vi "StartNewErrorLog.vi"(7 "LabVIEW Web Service Request":refnum<class "Web Request.lvclass">) -> ()   [LabVIEW 2018]
uses:
  <vilib>/wsapi/Web Request.lvclass
  CAEN globals.vi
panel:
  in  "error in (no error)":errorcluster
  # "Use the Web Service Request input terminal to call the VIs on the Web Services palette. Do not remove it from the connector pane unless you don't need access to the palette."
  # "Each additional control wired to the connector pane will be available as an input in the URL. To include an indicator in terminal-mode output (the default setting), it must also be wired to the connector pane."
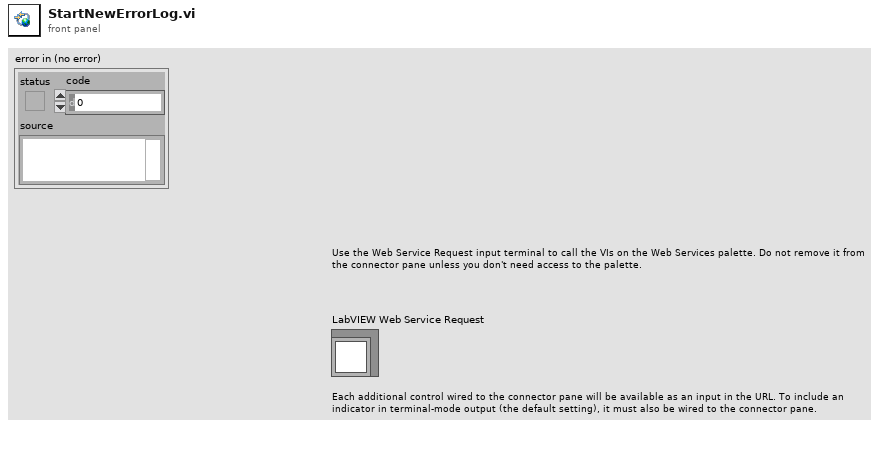
[diagram p1: front panel]
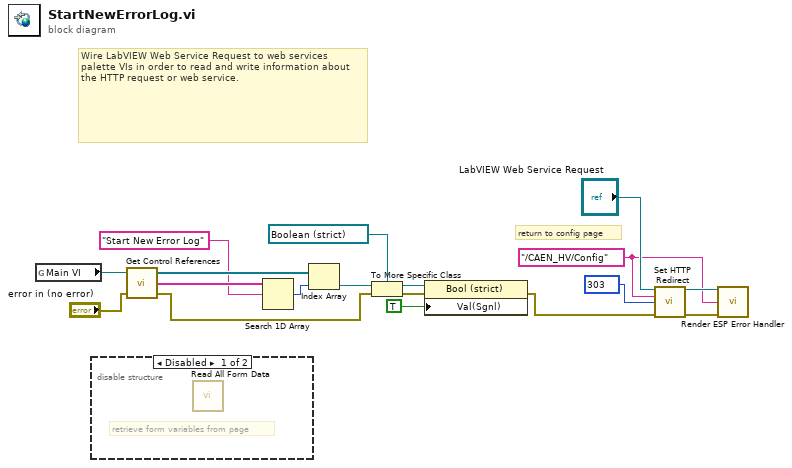
[diagram p0: block diagram]
diagram:
  w6 = 303 items=["100"=100, "101"=101, "200"=200, "201"=201, "202"=202, "203"=203, "204"=204, "205"=205, "206"=206, "300"=300, "301"=301, "302"=302, "303"=303, "304"=304, "305"=305, "306"=306, "307"=307, "400"=400, "401"=401, "402"=402, "403"=403, "404"=404, "405"=405, "406"=406, "407"=407, "408"=408, "409"=409, "410"=410, "411"=411, "412"=412, "413"=413, "414"=414, "415"=415, "416"=416, "417"=417, "500"=500, "501"=501, "502"=502, "503"=503, "504"=504, "505"=505] ("response code (307)")
  w1 = "/CAEN_HV/Config" ("redirect URL")
  # "return to config page"
  # "Wire LabVIEW Web Service Request to web services palette VIs in order to read and write information about the HTTP request or web service."
  n1 = global read "CAEN globals.vi" "Main VI"() -> (w18:refnum<vi>)
  n2 = disable-structure shown="Disabled" {
    frame Disabled {
      # "retrieve form variables from page"
      n3 = call <vilib>:"Read All Form Data.vi"() -> ()  [unwired: 11 in, 5 out]
    }
    frame Enabled {
    }
  }
  n4 = call "Get Control References.vi"("error in"="error in (no error)", "This vi"=w18) -> ("error out"=w8:errorcluster, "Control Names"=w17:string[], "Controls[]"=w16:refnum<vi>[])  [unwired: 1 in]
  n5 = Search 1D Array(1D array=w17, element="Start New Error Log" ("Label.Text")) -> (index of element=w11:i32)  [unwired: 1 in]
  n6 = Index Array(array=w16, index=w11) -> (element=w9:refnum<vi>)
  n7 = To More Specific Class(target class=refnum<vi> refnum ("replace all? (F)"), reference=w9, error in=w8) -> (specific class reference=w13:refnum<vi>, error out=w14:errorcluster)
  n8 = property class="Bool (strict)"(reference=w13, error in=w14, "Val(Sgnl)"=TRUE ("Value (Signaling)")) -> (error out=w3:errorcluster)  [unwired: 1 out]
  n9 = call <vilib>:"Set HTTP Redirect.vi"("LabVIEW Web Service Request"="LabVIEW Web Service Request", "redirect URL"=w1, "response code (307)"=w6, "error in (no error)"=w3) -> ("LabVIEW Web Service Request out"=w4:refnum<class "Web Request.lvclass">, "error out"=w5:errorcluster)  [unwired: 10 in]
  n10 = call "Render ESP Error Handler.vi"("LabVIEW Web Service Request"=w4, "Link"=w1, "error in (no error)"=w5) -> ()  [unwired: 11 in, 2 out]
